vi "TEST.vi"() -> ()   [LabVIEW 2009, in "Servo.lvlib"]
uses:
  Servo.lvlib
  PWM/PWM_Name.ctl
  PWM.lvlib
panel:
  in  "y":dbl
  out "Numeric":dbl
  in  "x":dbl min=-45.0 max=45.0
  in  "PWM":T1=1 items=["Invalid"=0, "PWM1"=1, "PWM2"=2, "PWM9"=9, "PWM10"=10]
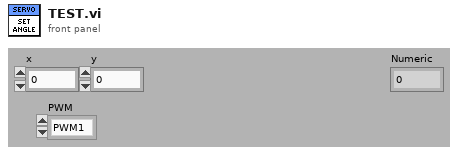
[diagram p1: front panel]
types:
  T1 = typedef "PWM.lvlib/PWM_Name.ctl" = u16
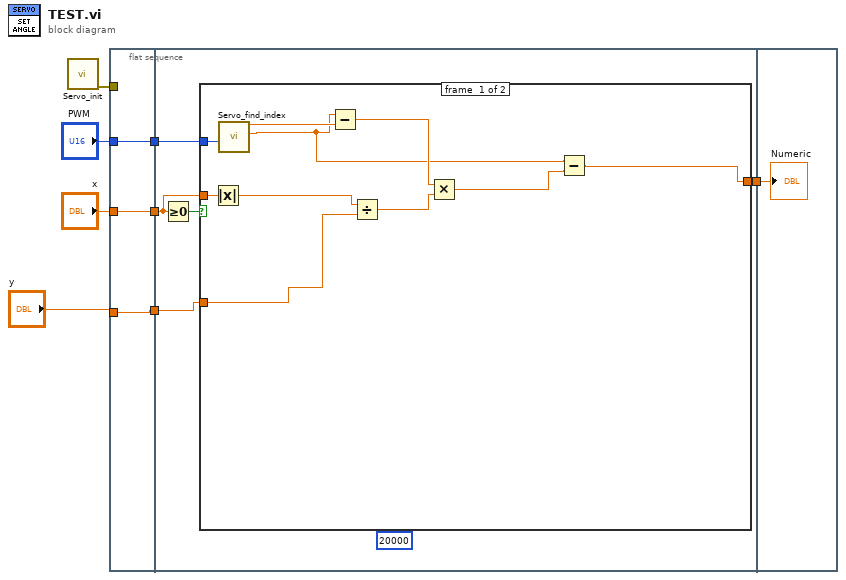
[diagram p0: block diagram]
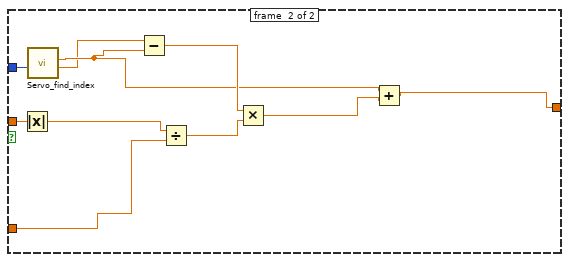
[diagram p2: hidden frame]
diagram:
  n1 = call "Servo_init.vi"() -> ("error out"=w7:errorcluster)  [unwired: 11 in]
  n2 = flat-sequence {
    tunnel: "PWM" -> [w10]
    tunnel: w7 -> [_]
    tunnel: "x" -> [w11]
    tunnel: [w11] -> w5
    tunnel: [w10] -> w4
    tunnel: "y" -> [w9]
    tunnel: [w9] -> w2
    tunnel: w5 -> [w15]
    tunnel: w4 -> [w14]
    tunnel: [w13] -> w3
    tunnel: w2 -> [w12]
    tunnel: w3 -> [w37]
    frame #0 {
    }
    frame #1 {
      (unwired) u32 20000 ("Period (uSec)")
      n3 = Greater Or Equal To 0?(x=w15) -> (x >= 0?=w16:bool)
      n4 = case shown="True" w16 {
        tunnel: w15 -> [w25 w35]
        tunnel: w14 -> [w26 w36]
        tunnel: [w22 w30] -> w13
        tunnel: w12 -> [w18 w32]
        frame #0 {
          n5 = Absolute Value(x=w25) -> (abs(x)=w19:dbl)
          n6 = call "Servo_find_index.vi"("PWM"=w26) -> ("value 2"=w20:dbl, "value"=w23:dbl)  [unwired: 7 in, 2 out]
          n7 = Subtract(x=w20, y=w23) -> (x-y=w24:dbl)
          n8 = Divide(x=w19, y=w18) -> (x/y=w17:dbl)
          n9 = Multiply(x=w24, y=w17) -> (x*y=w21:dbl)
          n10 = Subtract(x=w20, y=w21) -> (x-y=w22:dbl)
        }
        frame #1 {
          n11 = Absolute Value(x=w35) -> (abs(x)=w33:dbl)
          n12 = call "Servo_find_index.vi"("PWM"=w36) -> ("value 3"=w27:dbl, "value 2"=w28:dbl)  [unwired: 7 in, 2 out]
          n13 = Subtract(x=w27, y=w28) -> (x-y=w34:dbl)
          n14 = Divide(x=w33, y=w32) -> (x/y=w31:dbl)
          n15 = Multiply(x=w34, y=w31) -> (x*y=w29:dbl)
          n16 = Add(x=w28, y=w29) -> (x+y=w30:dbl)
        }
      }
    }
    frame #2 {
      "Numeric" <- w37
    }
  }
